vi "WaitForStop.vi"(3 "error in":errorcluster, 5 "Board ID":u8 min=1 max=32 step=1) -> (0 "error out 2":errorcluster, 1 "Stopped":bool, 2 "Bd ID Out":u8)   [LabVIEW 2022 SP3]
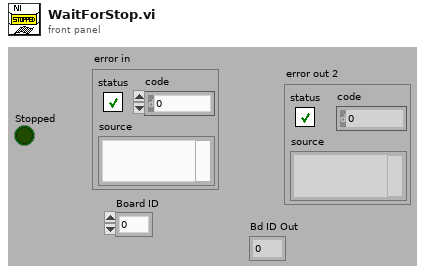
[diagram p1: front panel]
types:
  T1 = typedef "Bd Id Out" = u8
  T2 = cluster{"Reserved":bool, "Axis #1 Move Complete":bool, "Axis #2 Move Complete":bool, "Axis #3 Move Complete":bool, "Axis #4 Move Complete":bool, "Axis #5 Move Complete":bool, "Axis #6 Move Complete":bool, "Axis #7 Move Complete":bool, "Axis #8 Move Complete":bool, "Axis #9 MoveComplete":bool, "Axis #10 Move Complete":bool, "Axis #11 Move Complete":bool, "Axis #12 Move Complete":bool, "Status #13":bool, "Status #14":bool, "Status #15":bool}
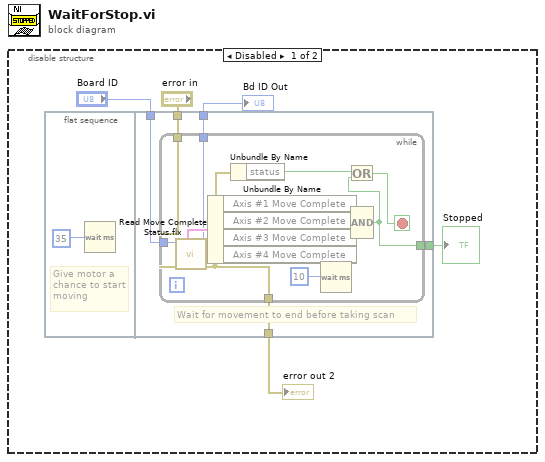
[diagram p0: block diagram]
diagram:
  n1 = disable-structure shown="Disabled" {
    frame Disabled {
      n2 = flat-sequence {
        tunnel: "Board ID" -> [w11]
        tunnel: [w10] -> w4
        tunnel: "error in" -> [w9]
        tunnel: [w8] -> w2
        tunnel: [w7] -> w1
        frame #0 {
          # "Give motor a chance to start moving"
          n3 = Wait (ms)(milliseconds to wait=35) -> ()  [unwired: 1 out]
        }
        frame #1 {
          # "Wait for movement to end before taking scan"
          n4 = while {
            tunnel: w11 -> [w19]
            tunnel: [w13] -> w10
            tunnel: w9 -> [w17]
            tunnel: [w15] -> w8
            tunnel: [w16] -> w7
            stop <- w12 stop-if-true
            n5 = call <vilib>:"Read Move Complete Status.flx"("error in (no error)"=w17, "Board ID"=w19) -> ("error out"=w15:errorcluster, "Bd ID Out"=w16:T1, "Move Complete Status"=w24:T2)  [unwired: 4 out]
            n6 = Unbundle By Name(w24) -> ("Axis #1 Move Complete"=w23:bool, "Axis #2 Move Complete"=w22:bool, "Axis #3 Move Complete"=w21:bool, "Axis #4 Move Complete"=w20:bool)
            n7 = Unbundle By Name(w15) -> ("status"=w14:bool)
            n8 = Wait (ms)(milliseconds to wait=10) -> ()  [unwired: 1 out]
            n9 = Compound Arithmetic op=AND(w23, w22, w21, w20) -> (w13:bool)
            n10 = Or(x=w14, y=w13) -> (x .or. y?=w12:bool)
          }
        }
      }
      "Stopped" <- w4
      "error out 2" <- w2
      "Bd ID Out" <- w1
    }
    frame Enabled {
    }
  }
